vi "ux with word.vi"() -> ()   [LabVIEW 2020]
panel:
  in  "Enum":enum16{"Device A", "Device B", "UBD5"}(ring)
  out "Array 3":string[](array[string])
  out "Length in bytes 3":i32
  out "if false  3":string
  out "Result of comparission 3":string
  out "Array 2":string[](array[string])
  out "Length in bytes 2":i32
  out "if false  2":string
  out "Result of comparission 2":string
  out "error out":errorcluster
  out "return value":string
  out "Array":string[](array[string])
  out "Length in bytes":i32
  out "if false":string
  out "Result of comparission":string
  out "Data In":u8[](array[numeric]) format="%.0x"
  out "Batch Length":i32
  out "Actual Bitrate kHz 2":i32=1000
  out "dup Cheetah Handle":i32
  out "Total Shifted Out":i32
  out "Actual Bitrate kHz":i32=1000
  out "error out 2":errorcluster
  in  "Rds per Sec":dbl=2000.0 max=2000000000.0
  out "SDO":u64[](array[numeric]) format="%x"
  in  "SCLK (kHz)":i32=2000 min=0
  out "Cheetah Handle":i32
  out "SDI":u64[](array[numeric]) format="%.0x"
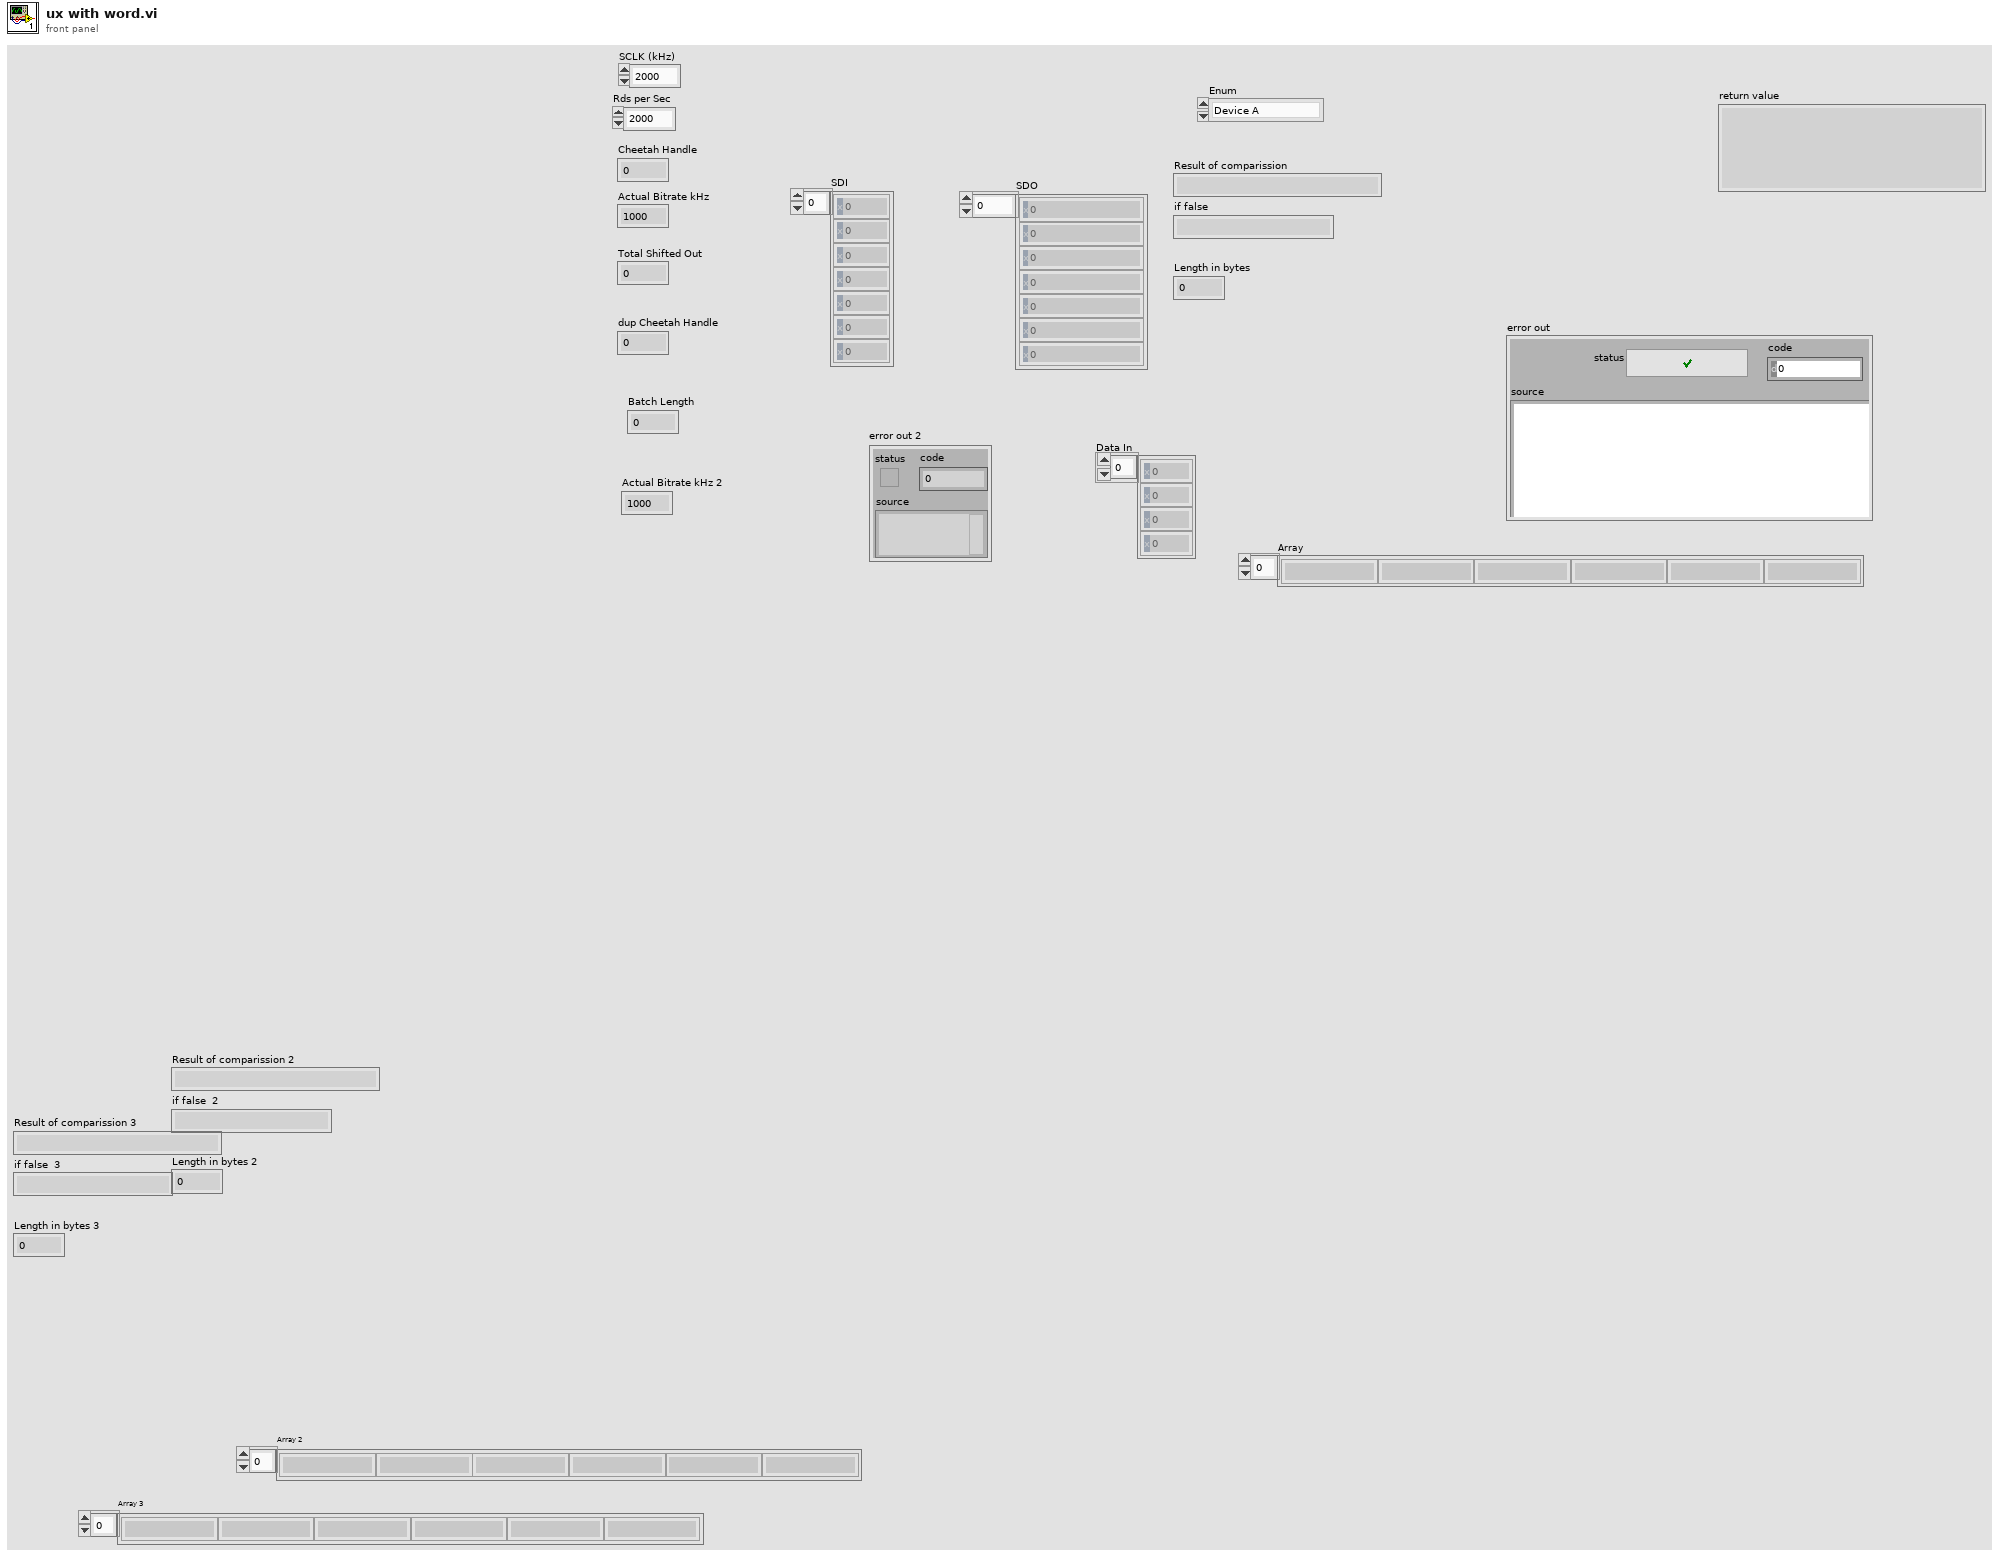
[diagram p1: front panel]
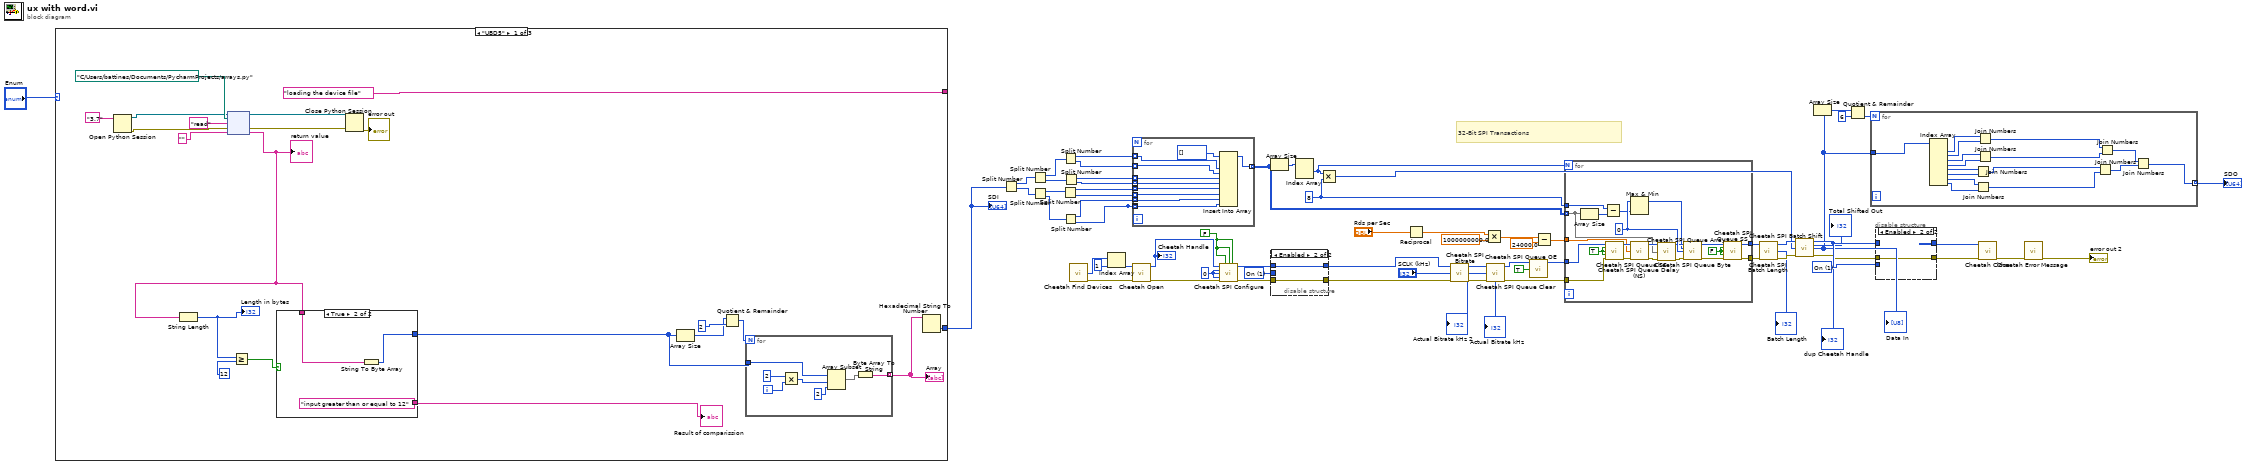
[diagram p0: block diagram]
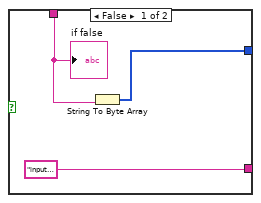
[diagram p2: hidden frame]
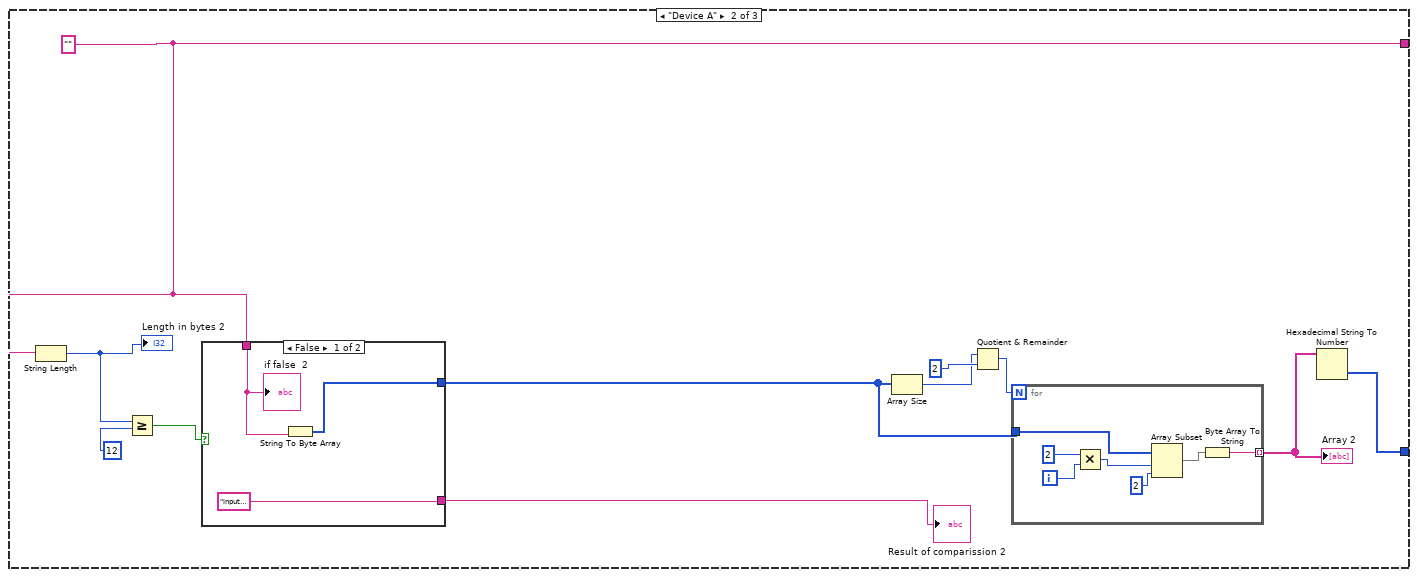
[diagram p3: hidden frame]
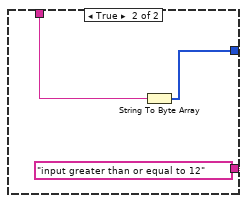
[diagram p4: hidden frame]
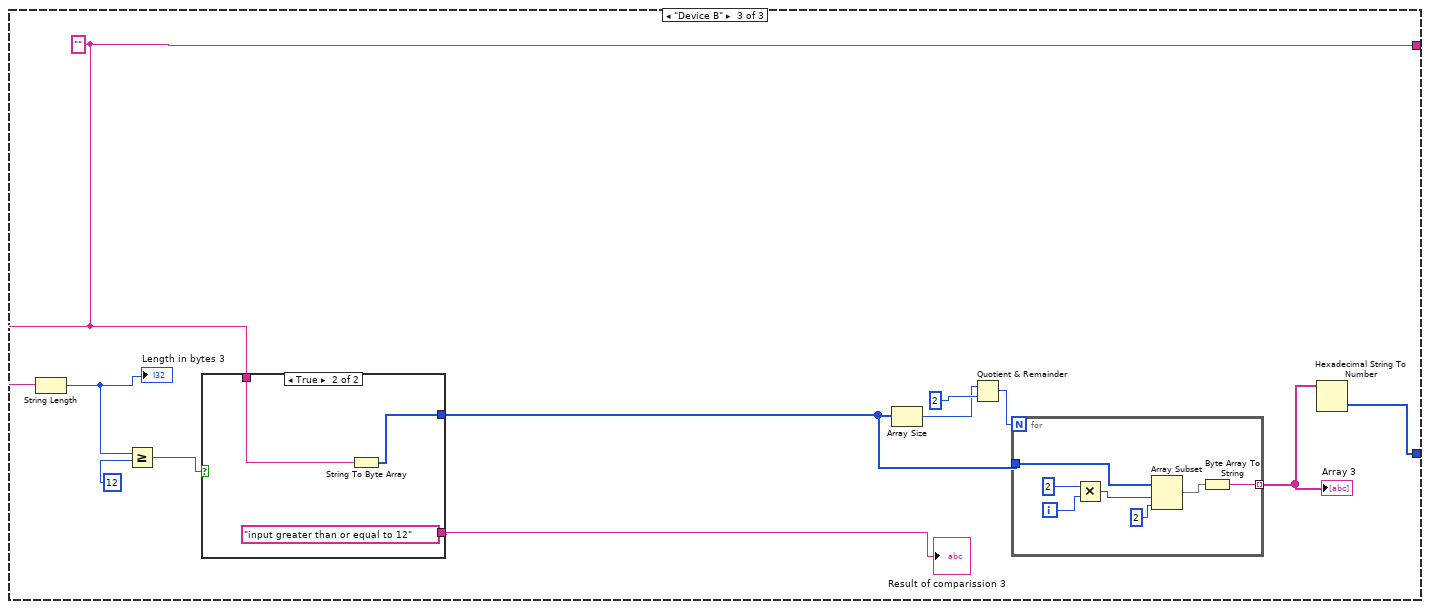
[diagram p5: hidden frame]
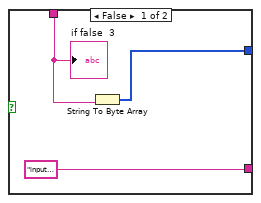
[diagram p6: hidden frame]
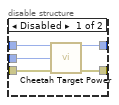
[diagram p7: hidden frame]
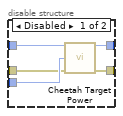
[diagram p8: hidden frame]
diagram:
  w21 = 8 ("y")
  w46 = u16 1 items=["Off", "On", "Query"] ("Requested Configuration (2: Query)")
  w47 = u16 1 items=["Off", "On", "Query"] ("Requested Configuration (2: Query)")
  w62 = FALSE
  w64 = 0
  # "32-Bit SPI Transactions"
  n1 = case shown="\"UBD5\"" "Enum" {
    tunnel: ["loading the device file" w102 w126] -> _
    tunnel: [w67 w101 w125] -> w2
    frame "UBD5" {
      n2 = Open Python Session(python version="3.7" ("Python version")) -> (session out=w78:refnum<k35>, error out=w79:errorcluster)  [unwired: 2 in]
      n3 = node(w78, path "C:/Users/battines/Documents/PycharmProjects/arrays.py" ("module path"), "read" ("function name"), w79, "") -> (w86:refnum<k35>, w87:errorcluster, w68:string)  [unwired: 2 out]
      "return value" <- w68
      n4 = String Length(string=w68) -> (length=w71:i32)
      "Length in bytes" <- w71
      n5 = Greater Or Equal?(x=w71, y=12) -> (x >= y?=w74:bool)
      n6 = case shown="True" w74 {
        tunnel: [w88 w93] -> w73
        tunnel: w68 -> [w89 w92]
        tunnel: ["input less than 12" "input greater than or equal to 12"] -> w72
        frame False {
          n7 = String To Byte Array(string=w89) -> (unsigned byte array=w88:u8[])
          "if false" <- w89
        }
        frame True {
          n8 = String To Byte Array(string=w92) -> (unsigned byte array=w93:u8[])
        }
      }
      "Result of comparission" <- w72
      n9 = Close Python Session(session in=w86, error in=w87) -> (11:→"error out":errorcluster)
      n10 = Array Size(array=w73) -> (size(s)=w69:i32)
      n11 = Quotient & Remainder(x=w69, y=2) -> (floor(x/y)=w77:i32)  [unwired: 1 out]
      n12 = for {
        N: w77 -> [_]
        tunnel: w73 -> [w100]
        tunnel: [w97] -> w76 mode=indexing
        i -> [w95]
        n13 = Multiply(x=2 ("y"), y=w95) -> (x*y=w99:i32)
        n14 = Array Subset(array=w100, index=w99, length=2) -> (w96:u8[])
        n15 = Byte Array To String(unsigned byte array=w96) -> (string=w97:string)
      }
      "Array" <- w76
      n16 = Hexadecimal String To Number(string=w76) -> (number=w67:u32[])  [unwired: 2 in, 1 out]
    }
    frame "Device A" {
      w102 = ""
      n17 = String Length(string=w102) -> (length=w105:i32)
      "Length in bytes 2" <- w105
      n18 = Greater Or Equal?(x=w105, y=12) -> (x >= y?=w108:bool)
      n19 = case shown="False" w108 {
        tunnel: [w112 w117] -> w107
        tunnel: w102 -> [w113 w116]
        tunnel: ["input less than 12" "input greater than or equal to 12"] -> w106
        frame False {
          n20 = String To Byte Array(string=w113) -> (unsigned byte array=w112:u8[])
          "if false  2" <- w113
        }
        frame True {
          n21 = String To Byte Array(string=w116) -> (unsigned byte array=w117:u8[])
        }
      }
      "Result of comparission 2" <- w106
      n22 = Array Size(array=w107) -> (size(s)=w103:i32)
      n23 = Quotient & Remainder(x=w103, y=2) -> (floor(x/y)=w111:i32)  [unwired: 1 out]
      n24 = for {
        N: w111 -> [_]
        tunnel: w107 -> [w124]
        tunnel: [w121] -> w110 mode=indexing
        i -> [w119]
        n25 = Multiply(x=2 ("y"), y=w119) -> (x*y=w123:i32)
        n26 = Array Subset(array=w124, index=w123, length=2) -> (w120:u8[])
        n27 = Byte Array To String(unsigned byte array=w120) -> (string=w121:string)
      }
      "Array 2" <- w110
      n28 = Hexadecimal String To Number(string=w110) -> (number=w101:u32[])  [unwired: 2 in, 1 out]
    }
    frame "Device B" {
      w126 = ""
      n29 = String Length(string=w126) -> (length=w129:i32)
      "Length in bytes 3" <- w129
      n30 = Greater Or Equal?(x=w129, y=12) -> (x >= y?=w132:bool)
      n31 = case shown="True" w132 {
        tunnel: [w136 w141] -> w131
        tunnel: w126 -> [w137 w140]
        tunnel: ["input less than 12" "input greater than or equal to 12"] -> w130
        frame False {
          n32 = String To Byte Array(string=w137) -> (unsigned byte array=w136:u8[])
          "if false  3" <- w137
        }
        frame True {
          n33 = String To Byte Array(string=w140) -> (unsigned byte array=w141:u8[])
        }
      }
      "Result of comparission 3" <- w130
      n34 = Array Size(array=w131) -> (size(s)=w127:i32)
      n35 = Quotient & Remainder(x=w127, y=2) -> (floor(x/y)=w135:i32)  [unwired: 1 out]
      n36 = for {
        N: w135 -> [_]
        tunnel: w131 -> [w148]
        tunnel: [w145] -> w134 mode=indexing
        i -> [w143]
        n37 = Multiply(x=2 ("y"), y=w143) -> (x*y=w147:i32)
        n38 = Array Subset(array=w148, index=w147, length=2) -> (w144:u8[])
        n39 = Byte Array To String(unsigned byte array=w144) -> (string=w145:string)
      }
      "Array 3" <- w134
      n40 = Hexadecimal String To Number(string=w134) -> (number=w125:u32[])  [unwired: 2 in, 1 out]
    }
  }
  "SDI" <- w2
  n41 = Split Number(x=w2) -> (hi(x)=w32:u16[], lo(x)=w31:u16[])
  n42 = Split Number(x=w32) -> (hi(x)=w9:u8[], lo(x)=w8:u8[])
  n43 = Split Number(x=w31) -> (hi(x)=w11:u8[], lo(x)=w10:u8[])
  n44 = Split Number(x=w11) -> (hi(x)=w15:u8[], lo(x)=w14:u8[])
  n45 = Split Number(x=w9) -> (hi(x)=w7:u8[], lo(x)=w6:u8[])
  n46 = Split Number(x=w10) -> (hi(x)=w13:u8[], lo(x)=w12:u8[])
  n47 = Split Number(x=w8) -> (hi(x)=w5:u8[], lo(x)=w4:u8[])
  n48 = call <instrlib>:"Cheetah Find Devices.vi"() -> ("Ports"=w65:u16[], "error out"=w61:errorcluster)  [unwired: 13 in, 1 out]
  n49 = Index Array(array=w65, index=1) -> (element=w53:u16)
  n50 = for {
    tunnel: w15 -> [w158] mode=indexing
    tunnel: [w157] -> w30 mode=indexing
    tunnel: w13 -> [w155] mode=indexing
    tunnel: w12 -> [_] mode=indexing
    tunnel: w12 -> [w154] mode=indexing
    tunnel: w14 -> [w153] mode=indexing
    tunnel: w7 -> [w152] mode=indexing
    tunnel: w6 -> [w151] mode=indexing
    tunnel: w5 -> [w150] mode=indexing
    tunnel: w4 -> [w149] mode=indexing
    n51 = Insert Into Array(array=u8[] [], new element #1=w152, new element #2=w151, new element #3=w150, new element #4=w149, new element #5=w158, new element #6=w153, new element #7=w155, new element #8=w154) -> (w157:u8[])  [unwired: 1 in]
  }
  n52 = call <instrlib>:"Cheetah Open.vi"("Port Number (0)"=w53, "error in (no error)"=w61) -> ("Cheetah Handle"=w58:i32, "error out"=w60:errorcluster)  [unwired: 12 in]
  "Cheetah Handle" <- w58
  n53 = call <instrlib>:"Cheetah SPI Configure.vi"("Cheetah Handle"=w58, "SS0 Active High? (False)"=w62, "SS1 Active High? (False)"=w62, "SS2 Active High? (False)"=w62, "Polarity (0: Rising/Falling)"=w64, "Phase (0: Sample/Setup)"=w64, "Bitorder (0: MSB)"=w64, "error in (no error)"=w60) -> ("dup Cheetah Handle"=w57:i32, "error out"=w59:errorcluster)  [unwired: 6 in]
  n54 = Array Size(array=w30) -> (size(s)=w45:i32[])
  n55 = disable-structure shown="Enabled" {
    disable-tunnel: w59 -> [w163 w164]
    disable-tunnel: w57 -> [w162 w165]
    disable-tunnel: [w161 w164] -> w56
    disable-tunnel: [w160 w165] -> w54
    disable-tunnel: w46 -> [w159 _]
    frame Disabled {
      n56 = call <instrlib>:"Cheetah Target Power.vi"("Cheetah Handle"=w162, "Requested Configuration (2: Query)"=w159, "error in (no error)"=w163) -> ("dup Cheetah Handle"=w160:i32, "error out"=w161:errorcluster)  [unwired: 10 in, 1 out]
    }
    frame Enabled {
    }
  }
  n57 = Index Array(array=w45) -> (element #1=w17:i32)  [unwired: 2 in, 1 out]
  n58 = Multiply(x=w17, y=w21) -> (x*y=w16:i32)
  n59 = Reciprocal(x="Rds per Sec") -> (1/x=w23:dbl)
  n60 = call <instrlib>:"Cheetah SPI Bitrate.vi"("Cheetah Handle"=w54, "Requested Bitrate kHz (1000)"="SCLK (kHz)", "error in (no error)"=w56) -> ("dup Cheetah Handle"=w52:i32, "Actual Bitrate kHz"=→"Actual Bitrate kHz" →"Actual Bitrate kHz 2":i32, "error out"=w51:errorcluster)  [unwired: 10 in]
  n61 = Multiply(x=w23, y=1000000000.0) -> (x*y=w26:dbl)
  n62 = call <instrlib>:"Cheetah SPI Queue Clear.vi"("Cheetah Handle"=w52, "error in (no error)"=w51) -> ("dup Cheetah Handle"=w44:i32, "error out"=w63:errorcluster)  [unwired: 12 in]
  n63 = call <instrlib>:"Cheetah SPI Queue OE.vi"("Cheetah Handle"=w44, "Output Enable (on)"=TRUE) -> ("dup Cheetah Handle"=w43:i32)  [unwired: 12 in, 1 out]
  n64 = Subtract(x=w26, y=24000.0) -> (x-y=w24:dbl)
  n65 = for {
    N: w17 -> [_]
    tunnel: w63 -> [w172]
    tunnel: w43 -> [w173]
    tunnel: w30 -> [w174] mode=indexing
    tunnel: [w171] -> w41
    tunnel: [w170] -> w40
    tunnel: w24 -> [w167]
    tunnel: w21 -> [w168]
    w178 = FALSE
    w181 = 0
    w169 = TRUE
    n66 = Array Size(array=w174) -> (size(s)=w175:i32)
    n67 = Subtract(x=w168, y=w175) -> (x-y=w179:i32)
    n68 = call <instrlib>:"Cheetah SPI Queue SS.vi"("Cheetah Handle"=w173, "SS0 Assert? (True)"=w169, "SS1 Assert? (True)"=w169, "SS2 Assert? (True)"=w169, "error in (no error)"=w172) -> ("dup Cheetah Handle"=w186:i32, "error out"=w185:errorcluster)  [unwired: 9 in]
    n69 = Max & Min(x=w181, y=w179) -> (max(x,y)=w166:i32)  [unwired: 1 out]
    n70 = call <instrlib>:"Cheetah SPI Queue Delay (NS).vi"("Cheetah Handle"=w186, "Delay NS (1000)"=w167, "error in (no error)"=w185) -> ("dup Cheetah Handle"=w184:i32, "error out"=w183:errorcluster)  [unwired: 10 in, 1 out]
    n71 = call <instrlib>:"Cheetah SPI Queue Array.vi"("Cheetah Handle"=w184, "Data Out (none)"=w174, "error in (no error)"=w183) -> ("dup Cheetah Handle"=w180:i32, "error out"=w182:errorcluster)  [unwired: 11 in]
    n72 = call <instrlib>:"Cheetah SPI Queue Byte.vi"("Cheetah Handle"=w180, "Byte Count (1)"=w166, "Byte Value (0x00)"=w181, "error in (no error)"=w182) -> ("dup Cheetah Handle"=w177:i32, "error out"=w176:errorcluster)  [unwired: 10 in]
    n73 = call <instrlib>:"Cheetah SPI Queue SS.vi"("Cheetah Handle"=w177, "SS0 Assert? (True)"=w178, "SS1 Assert? (True)"=w178, "SS2 Assert? (True)"=w178, "error in (no error)"=w176) -> ("dup Cheetah Handle"=w170:i32, "error out"=w171:errorcluster)  [unwired: 9 in]
  }
  n74 = call <instrlib>:"Cheetah SPI Batch Length.vi"("Cheetah Handle"=w40, "error in (no error)"=w41) -> ("dup Cheetah Handle"=w39:i32, "Batch Length"=→"Batch Length":i32, "error out"=w38:errorcluster)  [unwired: 11 in]
  n75 = call <instrlib>:"Cheetah SPI Batch Shift.vi"("Cheetah Handle"=w39, "Max Bytes to Retrieve (256)"=w16, "error in (no error)"=w38) -> ("dup Cheetah Handle"=w37:i32, "Total Shifted Out"=→"Total Shifted Out":i32, "Data In"=w18:u8[], "error out"=w29:errorcluster)  [unwired: 9 in]
  "dup Cheetah Handle" <- w37
  "Data In" <- w18
  n76 = Array Size(array=w18) -> (size(s)=w36:i32)
  n77 = Quotient & Remainder(x=w36, y=6) -> (floor(x/y)=w34:i32)  [unwired: 1 out]
  n78 = for {
    N: w34 -> [_]
    tunnel: w18 -> [w201]
    tunnel: [w200] -> w33 mode=indexing
    n79 = Index Array(array=w201) -> (element #1=w190:u8, element #2=w189:u8, element #3=w188:u8, element #4=w187:u8, element #5=w199:u8, element #6=w198:u8, element #7=w197:u8, element #8=w196:u8)  [unwired: 8 in]
    n80 = Join Numbers(hi=w199, lo=w198) -> ((hi.lo)=w195:u16)
    n81 = Join Numbers(hi=w197, lo=w196) -> ((hi.lo)=w194:u16)
    n82 = Join Numbers(hi=w190, lo=w189) -> ((hi.lo)=w193:u16)
    n83 = Join Numbers(hi=w188, lo=w187) -> ((hi.lo)=w192:u16)
    n84 = Join Numbers(hi=w195, lo=w194) -> ((hi.lo)=w202:u32)
    n85 = Join Numbers(hi=w193, lo=w192) -> ((hi.lo)=w191:u32)
    n86 = Join Numbers(hi=w191, lo=w202) -> ((hi.lo)=w200:u64)
  }
  "SDO" <- w33
  n87 = disable-structure shown="Enabled" {
    disable-tunnel: [w207 _] -> w50
    disable-tunnel: [w206 w208] -> w49
    disable-tunnel: w47 -> [w205 _]
    disable-tunnel: w37 -> [w204 _]
    disable-tunnel: w29 -> [w203 w208]
    frame Disabled {
      n88 = call <instrlib>:"Cheetah Target Power.vi"("Cheetah Handle"=w204, "Requested Configuration (2: Query)"=w205, "error in (no error)"=w203) -> ("dup Cheetah Handle"=w207:i32, "error out"=w206:errorcluster)  [unwired: 10 in, 1 out]
    }
    frame Enabled {
    }
  }
  n89 = call <instrlib>:"Cheetah Close.vi"("Cheetah Handle"=w50, "error in (no error)"=w49) -> ("error out"=w48:errorcluster)  [unwired: 12 in, 1 out]
  n90 = call <instrlib>:"Cheetah Error Message.vi"("error in (no error)"=w48) -> ("error out"=→"error out 2":errorcluster)  [unwired: 10 in, 4 out]
